vi "Enqueue Message.vi"(9 "data (empty)":variant, 10 "message":string) -> (3 "channel":T1)   [LabVIEW 2019, in "Message Queue.lvlib"]
doc: "This VI puts messages into the messenger channel."
uses:
  03.3 Queued Message Handler/support/Message Queue/Message Queue.lvlib
  <extravilib>/ChannelInstances/Messenger-t'Message Queue.lvlib-Message Cluster.ctl'/))Channel.ctl
  Message Cluster.ctl
  <extravilib>/ChannelInstances/Messenger-t'Message Queue.lvlib-Message Cluster.ctl'/Write With Abort.vi
  <resource>/Channels/Messenger/Write With Abort.vi
  <extravilib>/ChannelInstances/Messenger-t'Message Queue.lvlib-Message Cluster.ctl'/Wrapper.lvclass
  C:/Program Files/National Instruments/LabVIEW 2019/vi.lib/ChannelSupport/Channel Message/Channel Message.lvclass
  <extravilib>/ChannelInstances/Messenger-t'Message Queue.lvlib-Message Cluster.ctl'/Wrap.vi
  <resource>/Channels/Messenger/Endpoint.vi
  <extravilib>/ChannelInstances/Messenger-t'Message Queue.lvlib-Message Cluster.ctl'.lvlib
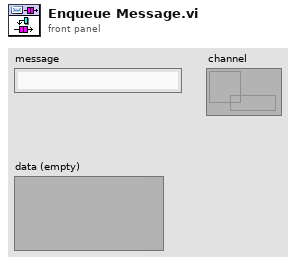
[diagram p1: front panel]
types:
  T1 = typedef "Messenger-t'Message Queue.lvlib-Message Cluster.ctl'.lvlib/))Channel.ctl" = refnum<queue>
  T2 = typedef "Message Queue.lvlib/Message Cluster.ctl" = cluster{"Message":string, "Message Data":variant}
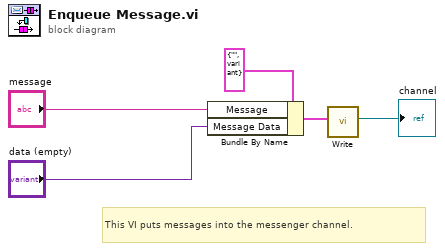
[diagram p0: block diagram]
diagram:
  # "This VI puts messages into the messenger channel."
  n1 = Bundle By Name(cluster=T2 {"Message"="", "Message Data"=variant} ("Message Cluster"), "Message"="message", "Message Data"="data (empty)") -> (w1:T2)
  n2 = call <extravilib>:"Write.vi"("element"=w1) -> ("channel"=→"channel":T1)  [unwired: 8 in, 2 out]
